vi "TCL_Simulated Temperature Control.vi"() -> ()   [LabVIEW 2012]
uses:
  SupportVIs.llb/TS_RT-globalvar.vi
  SupportVIs.llb/TS_RT-Integrator.vi
  SupportVIs.llb/TS_RT-PID.vi
panel:
  in  "PID gains":T1={"proportional gain (Kc)"=1.0, "integral time (Ti, min)"=2.0, "derivative time (Td, min)"=0.0} {"derivative time (Td, min)" format="%.3f"; "integral time (Ti, min)" format="%.3f"; "proportional gain (Kc)" format="%.3f"}
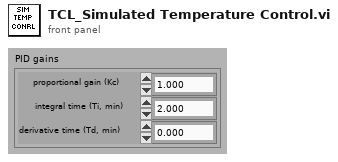
[diagram p1: front panel]
types:
  T1 = cluster{"proportional gain (Kc)":dbl, "integral time (Ti, min)":dbl, "derivative time (Td, min)":dbl}
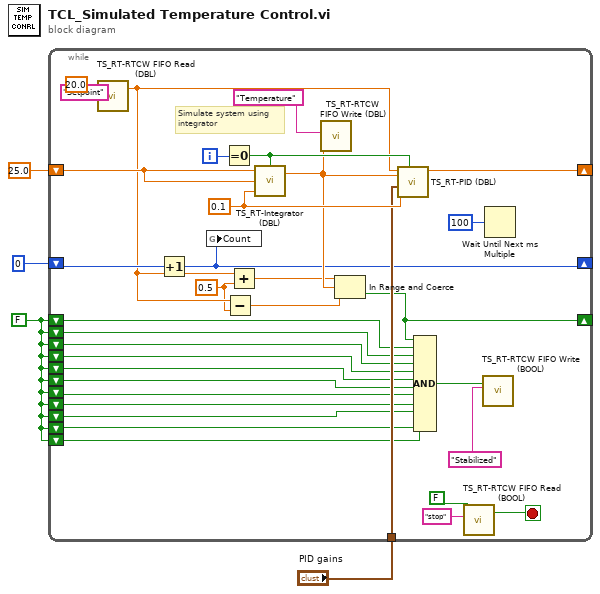
[diagram p0: block diagram]
diagram:
  w1 = FALSE
  n1 = while {
    shift-right: [w33] -> _
    shift-left: 25.0 ("output") -> [w38]
    tunnel: "PID gains" -> [w31]
    shift-right: [w15] -> _
    shift-left: 0 -> [w30]
    shift-right: [w29] -> _
    shift-left: w1 -> [w28]
    shift-left: w1 -> [w27]
    shift-left: w1 -> [w26]
    shift-left: w1 -> [w25]
    shift-left: w1 -> [w24]
    shift-left: w1 -> [w23]
    shift-left: w1 -> [w22]
    shift-left: w1 -> [w21]
    shift-left: w1 -> [w20]
    shift-left: w1 -> [w19]
    shift-left: w1 -> [w18]
    i -> [w37]
    stop <- w32 stop-if-true
    w7 = 0.5 ("y")
    w35 = 0.1 ("dt")
    # "Simulate system using\nintegrator"
    n2 = call "TS_RT-RTCW FIFO Read (DBL).vi"("name (unnamed)"="Setpoint", "init"=20.0) -> ("output"=w8:dbl)  [unwired: 1 in, 8 out]
    n3 = Increment(x=w30) -> (x+1=w15:i32)
    n4 = global write "TS_RT-globalvar.vi" "Count"(w15) -> ()
    n5 = Equal To 0?(x=w37) -> (x = 0?=w34:bool)
    n6 = Subtract(x=w8, y=w7) -> (x-y=w6:dbl)
    n7 = Add(x=w8, y=w7) -> (x+y=w5:dbl)
    n8 = call-poly "TS_RT-Integrator (DBL).vi"("initialize"=w34, "dt"=w35, "initial condition"=w38, "input point"=w38) -> ("output point"=w16:dbl)  [unwired: 1 out]
    n9 = call "TS_RT-RTCW FIFO Write (DBL).vi"("name (unnamed)"="Temperature", "input"=w16) -> ()  [unwired: 2 in, 8 out]
    n10 = In Range and Coerce(upper limit=w5, x=w16, lower limit=w6) -> (In Range?=w29:bool)  [unwired: 1 out]
    n11 = call-poly "TS_RT-PID (DBL).vi"("reinitialize? (F)"=w34, "dt (s)"=w35, "PID gains"=w31, "process variable"=w16, "setpoint"=w8) -> ("output"=w33:dbl)  [unwired: 1 in, 5 out]
    n12 = Compound Arithmetic op=AND(w29, w28, w27, w26, w25, w24, w23, w22, w21, w20, w19, w18) -> (w17:bool)
    n13 = call "TS_RT-RTCW FIFO Read (BOOL).vi"("name (unnamed)"="stop", "init"=FALSE) -> ("output"=w32:bool)  [unwired: 1 in, 8 out]
    n14 = call "TS_RT-RTCW FIFO Write (BOOL).vi"("name (unnamed)"="Stabilized", "input"=w17) -> ()  [unwired: 2 in, 8 out]
    n15 = Wait Until Next ms Multiple(millisecond multiple=u32 100) -> ()  [unwired: 1 out]
  }
